vi "Test MQTT-4.7.3-3.vi"(8 "error in (no error)":errorcluster) -> (0 "error out":errorcluster)   [LabVIEW 2013]
uses:
  <vilib>/addons/_JKI Toolkits/Caraya/classes/Test/Test.lvclass
  source/TopicFilter/TopicFilter.lvclass
  <vilib>/addons/_JKI Toolkits/Caraya/classes/Assert/Assert.lvclass
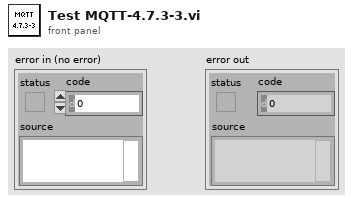
[diagram p1: front panel]
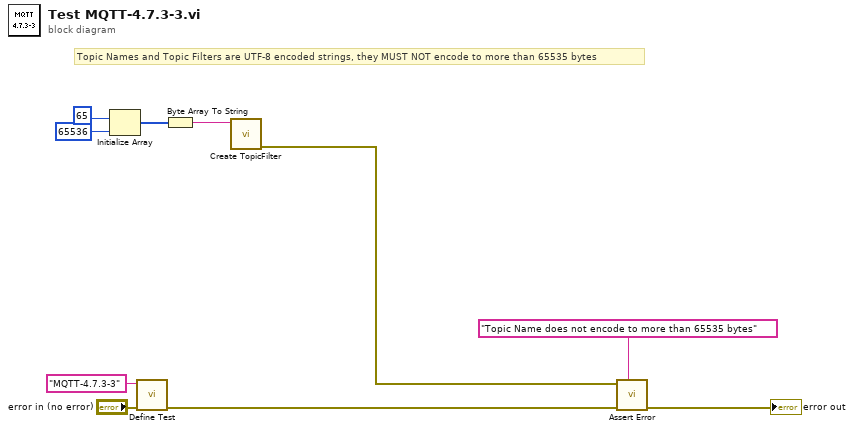
[diagram p0: block diagram]
diagram:
  # "Topic Names and Topic Filters are UTF-8 encoded strings, they MUST NOT encode to more than 65535 bytes"
  n1 = Initialize Array(u8 65, 65536 ("dimension size")) -> (w2:u8[])
  n2 = call <vilib>:"Define Test.vi"("error in (no error)"="error in (no error)", "Label (VI Title)"="MQTT-4.7.3-3") -> ("error out"=w7:errorcluster)  [unwired: 9 in]
  n3 = Byte Array To String(unsigned byte array=w2) -> (string=w4:string)
  n4 = call "Create TopicFilter.vi"("Topic Filter"=w4) -> ("error out"=w5:errorcluster)  [unwired: 9 in, 1 out]
  n5 = call <vilib>:"Assert Error.vi"("Label"="Topic Name does not encode to more than 65535 bytes", "error in (no error)"=w7, "Error?"=w5) -> ("error out"=→"error out":errorcluster)  [unwired: 8 in]
